vi "tanh_v1.1.vi"(1 "x":T1) -> (0 "y":T1)   [LabVIEW 2020]
uses:
  <vilib>/Analysis/Matrix/Datatypes/RealMatrix.ctl
  <vilib>/Analysis/Matrix/Numeric/Conversions/Matrix To Array - RM.vi
  <vilib>/Analysis/Matrix/Numeric/Conversions/Array To Matrix - RA.vi
  <vilib>/Analysis/Matrix/NI_Matrix.lvlib
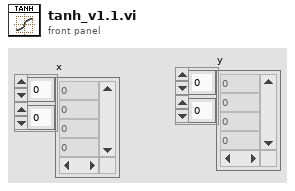
[diagram p1: front panel]
types:
  T1 = typedef "NI_Matrix.lvlib/RealMatrix.ctl" = dbl[][]
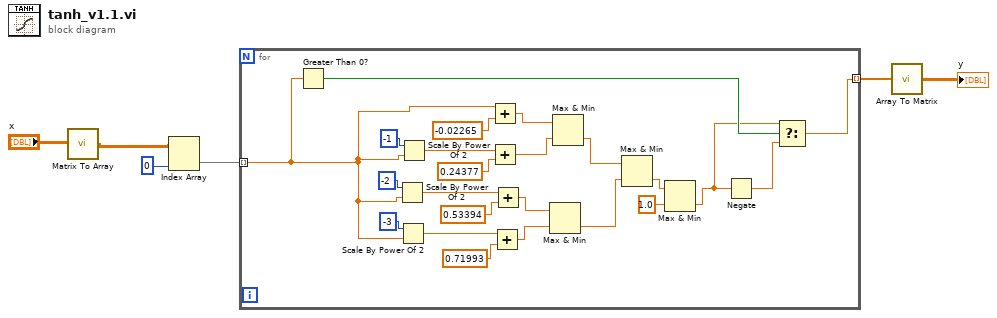
[diagram p0: block diagram]
diagram:
  n1 = call-poly <vilib>:"Matrix To Array.vi"("Real Matrix"="x") -> ("Real 2D Array"=w1:dbl[][])
  n2 = Index Array(array=w1, index (col)=0) -> (element=w5:dbl[])  [unwired: 1 in]
  n3 = for {
    tunnel: w5 -> [w11] mode=indexing
    tunnel: [w7] -> w4 mode=indexing
    n4 = Greater Than 0?(x=w11) -> (x > 0?=w10:bool)
    n5 = Scale By Power Of 2(n=-2, x=w11) -> (x*2^n=w22:dbl)
    n6 = Scale By Power Of 2(n=-3, x=w11) -> (x*2^n=w14:dbl)
    n7 = Scale By Power Of 2(n=-1, x=w11) -> (x*2^n=w21:dbl)
    n8 = Add(x=w11, y=-0.02265) -> (x+y=w20:dbl)
    n9 = Add(x=w21, y=0.24377) -> (x+y=w19:dbl)
    n10 = Add(x=w14, y=0.71993) -> (x+y=w17:dbl)
    n11 = Add(x=w22, y=0.53394) -> (x+y=w18:dbl)
    n12 = Max & Min(x=w18, y=w17) -> (min(x,y)=w15:dbl)  [unwired: 1 out]
    n13 = Max & Min(x=w20, y=w19) -> (min(x,y)=w16:dbl)  [unwired: 1 out]
    n14 = Max & Min(x=w16, y=w15) -> (min(x,y)=w12:dbl)  [unwired: 1 out]
    n15 = Max & Min(x=w12, y=1.0) -> (min(x,y)=w9:dbl)  [unwired: 1 out]
    n16 = Negate(x=w9) -> (-x=w8:dbl)
    n17 = Select(t=w9, s=w10, f=w8) -> (s? t:f=w7:dbl)
  }
  n18 = call-poly <vilib>:"Array To Matrix.vi"("Real 1D Array"=w4) -> ("Real Matrix (Column Vector)"=→"y":T1)
